vi "Create Error.vi"(7 "Call Chain (F)":bool, 8 "MultiErrors in":refnum<class "MultiErrors.lvclass">, 10 "Message":string, 11 "Code":i32=1) -> (0 "MultiErrors out":refnum<class "MultiErrors.lvclass">)   [LabVIEW 2020, in "Volatus.lvlib" / "MultiErrors.lvclass"]
uses:
  MultiErrors.lvclass
  MultiError Entry.ctl
  MultiErrors.lvclass/MultiErrors.ctl
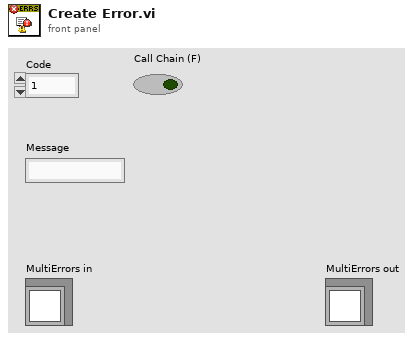
[diagram p1: front panel]
types:
  T1 = typedef "Volatus.lvlib/MultiErrors.lvclass/MultiError Entry.ctl" = cluster{"Context":string[], "Message":string, "Code":i32, "Call Chain":string[]}
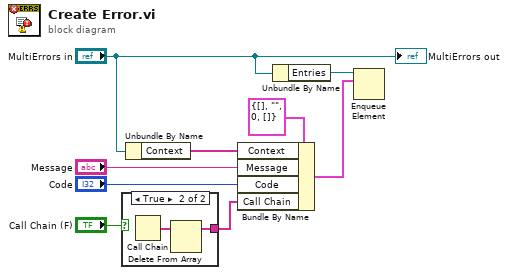
[diagram p0: block diagram]
diagram:
  n1 = case shown="True" "Call Chain (F)" {
    tunnel: [_ w10] -> w4
    frame False {
    }
    frame True {
      n2 = Call Chain() -> (call chain=w11:string[])
      n3 = Delete From Array(array=w11) -> (array with subset deleted=w10:string[])  [unwired: 2 in, 1 out]
    }
  }
  n4 = Unbundle By Name("MultiErrors in") -> ("Context"=w8:string[])
  n5 = Bundle By Name(cluster=T1 {"Context"=[], "Message"="", "Code"=0, "Call Chain"=[]} ("MultiError Entry"), "Context"=w8, "Message"="Message", "Code"="Code", "Call Chain"=w4) -> (w1:T1)
  n6 = Unbundle By Name("MultiErrors in") -> ("Entries"=w2:refnum<queue>)
  n7 = Enqueue Element(queue=w2, element=w1) -> ()  [unwired: 2 in, 3 out]
  "MultiErrors out" <- "MultiErrors in"
